vi "Finish.vi"   [LabVIEW 2018]
doc: "This VI is called just before exiting. It is expected to close I/O refnum, save collected data, etc."
uses:
  Global_Variables/Refnum_Names.vi
  <vilib>/Rock Robotics/WPI/Utilities/WPI_GetSetVariantRefNum.vi
types:
  T1 = typedef "WPI_JoystickDevRef.ctl" = cluster{"Device":T2}
  T2 = typedef "WPI_JoystickDeviceEnum.ctl" = enum16{"USB 0", "USB 1", "USB 2", "USB 3", "USB 4", "USB 5"}
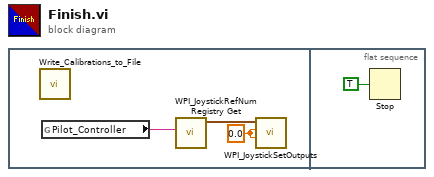
[diagram p0: block diagram]
diagram:
  n1 = flat-sequence {
    frame #0 {
      w2 = sgl 0.0 ("Left Rumble")
      n2 = call "Write_Calibrations_to_File.vi"() -> ()  [unwired: 12 in]
      n3 = global read "Refnum_Names.vi" "Pilot_Controller"() -> (w1:string)
      n4 = call <vilib>:"WPI_JoystickRefNum Registry Get.vi"("refnum name"=w1) -> ("JoystickDevRef"=w3:T1)  [unwired: 9 in, 1 out]
      n5 = call <vilib>:"WPI_JoystickSetOutputs.vi"("Right Rumble"=w2, "Left Rumble"=w2, "JoystickDevRef"=w3) -> ()  [unwired: 7 in, 2 out]
    }
    frame #1 {
      n6 = Stop(stop? (T)=TRUE) -> ()
    }
  }
